vi "FT_Set_Bit_Mode.vi"(1 "Bit Mode":u8(ring) items=["Reset Bit Mode"=0, "Asynchronous Bit Bang"=1, "MPSSE"=2, "Synchronous Bit Bang"=4, "MCU Host Bus Emulation"=8, "Fast Opto-Isolated Serial"=16, "CBUS Bit Bang"=32, "Single Channel 245 Synchronous FIFO"=64], 2 "Bit Mode Mask":u8 format="%x", 3 "Handle":u32) -> (0 "FT_Status":u32(ring) items=["FT_OK", "FT_INVALID_HANDLE", "FT_DEVICE_NOT_FOUND", "FT_DEVICE_NOT_OPENED", "FT_IO_ERROR", "FT_INSUFFICIENT_RESOURCES", "FT_INVALID_PARAMETER", "FT_INVALID_BAUD_RATE", "FT_DEVICE_NOT_OPENED_FOR_ERASE", "FT_DEVICE_NOT_OPENED_FOR_WRITE", "FT_FAILED_TO_WRITE_DEVICE", "FT_EEPROM_READ_FAILED", "FT_EEPROM_WRITE_FAILED", "FT_EEPROM_ERASE_FAILED", "FT_EEPROM_NOT_PRESENT", "FT_EEPROM_NOT_PROGRAMMED", "FT_INVALID_ARGS", "FT_NOT_SUPPORTED", "FT_OTHER_ERROR"])   [LabVIEW 2012]
uses:
  FTD2XX.dll
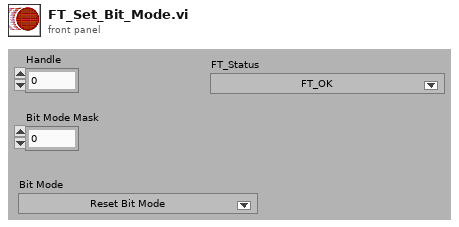
[diagram p1: front panel]
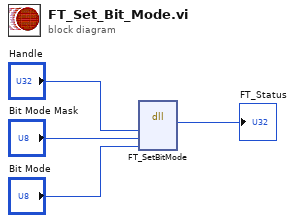
[diagram p0: block diagram]
diagram:
  n1 = dll-call lib="FTD2XX.dll" fn="FT_SetBitMode"("Handle"="Handle", "Mask"="Bit Mode Mask", "Enable"="Bit Mode") -> ("FT_Status"=→"FT_Status":u32)  [unwired: 6 in, 2 out]
